vi "GET.vi"(6 "timeout":i32=10000, 7 "output file":path, 8 "error in":errorcluster, 10 "url":string, 11 "http-client in":refnum<class "http-client.lvclass">) -> (0 "error out":errorcluster, 1 "body":string, 2 "headers":string, 3 "http-client out":refnum<class "http-client.lvclass">)   [LabVIEW 2020, in "REST Client.lvlib" / "http-client.lvclass"]
uses:
  http-client.lvclass
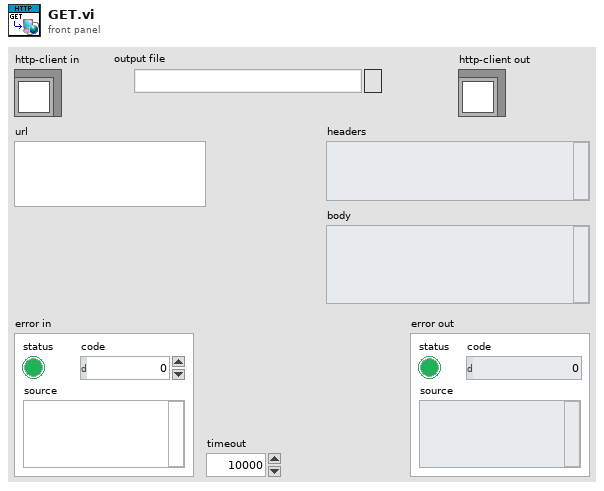
[diagram p1: front panel]
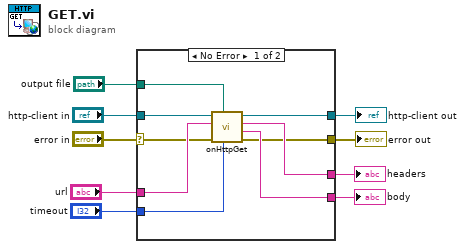
[diagram p0: block diagram]
diagram:
  n1 = case shown="No Error" "error in" {
    selector: "error in" -> [w11 w20]
    tunnel: [w10 w20] -> w8
    tunnel: [w16 w19] -> w6
    tunnel: "http-client in" -> [w17 w19]
    tunnel: [w15 _] -> w5
    tunnel: "url" -> [w12 _]
    tunnel: "timeout" -> [w13 _]
    tunnel: "output file" -> [w18 _]
    tunnel: [w14 _] -> w1
    frame No Error {
      n2 = call-dynamic "onHttpGet.vi"("timeout"=w13, "output file"=w18, "error in"=w11, "url"=w12, "http-method in"=w17) -> ("error out"=w10:errorcluster, "body"=w14:string, "headers"=w15:string, "http-method out"=w16:refnum<class "http-client.lvclass">)  [unwired: 3 in]
    }
    frame Error {
    }
  }
  "error out" <- w8
  "http-client out" <- w6
  "headers" <- w5
  "body" <- w1
